vi "Byte_to_bit.vi"(6 "Error In":errorcluster, 7 "BYTE":string, 8 "Array of byte":u8[](array[numeric])) -> (0 "Error Out":errorcluster, 1 "Arrray of bit (str)":u8[](array[numeric]), 2 "Arrray of bit":u8[](array[numeric]))   [LabVIEW 2019]
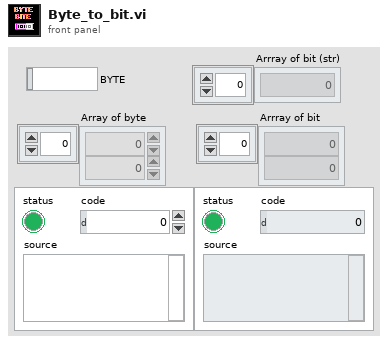
[diagram p1: front panel]
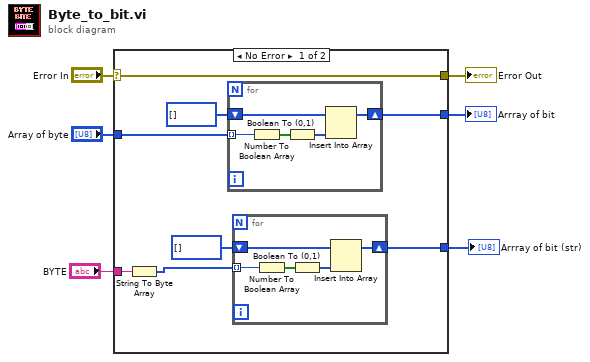
[diagram p0: block diagram]
diagram:
  n1 = case shown="No Error" "Error In" {
    selector: "Error In" -> [w11 w25]
    tunnel: [w13 _] -> w6
    tunnel: "Array of byte" -> [w14 _]
    tunnel: [w11 w25] -> w3
    tunnel: [w10 _] -> w2
    tunnel: "BYTE" -> [w8 _]
    frame No Error {
      n2 = String To Byte Array(string=w8) -> (unsigned byte array=w7:u8[])
      n3 = for {
        tunnel: w14 -> [w24] mode=indexing
        shift-right: [w21] -> w13
        shift-left: u8[] [] -> [w20]
        n4 = Number To Boolean Array(number=w24) -> (Boolean array=w23:bool[])
        n5 = Boolean To (0,1)(Boolean=w23) -> (0, 1=w22:i16[])
        n6 = Insert Into Array(array=w20, new element=w22) -> (w21:u8[])  [unwired: 1 in]
      }
      n7 = for {
        tunnel: w7 -> [w19] mode=indexing
        shift-right: [w16] -> w10
        shift-left: u8[] [] -> [w15]
        n8 = Number To Boolean Array(number=w19) -> (Boolean array=w18:bool[])
        n9 = Boolean To (0,1)(Boolean=w18) -> (0, 1=w17:i16[])
        n10 = Insert Into Array(array=w15, new element=w17) -> (w16:u8[])  [unwired: 1 in]
      }
    }
    frame Error {
    }
  }
  "Arrray of bit" <- w6
  "Error Out" <- w3
  "Arrray of bit (str)" <- w2
